vi "마이크로세크 카운터.vi"() -> ()   [LabVIEW 2018]
uses:
  <vilib>/DAQmx/read.llb/DAQmx Read (Counter DBL 1Chan 1Samp).vi
  <vilib>/DAQmx/create/channels.llb/DAQmx Create Channel (CI-Count Edges).vi
  <vilib>/DAQmx/miscellaneous.llb/DAQmx Fill In Error Info.vi
panel:
  out "Elapsed time [s]":dbl
  in  "Input Frequency [Hz]":dbl format="%0.2f"
  out "data 2":dbl caption="데이터" format="%0.2f"
  in  "정지 버튼":bool
  in  "edge":i32(ring)=10280 caption="에지" items=["상승"=10280, "하강"=10171]
  in  "count direction":i32(ring)=10128 caption="카운트 방향" items=["카운트 업"=10128, "카운트 다운"=10124, "외부 컨트롤"=10326]
  in  "initial count":u32 caption="초기 카운트"
  in  "counter":tag caption="카운터"
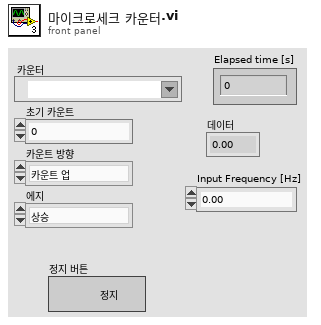
[diagram p1: front panel]
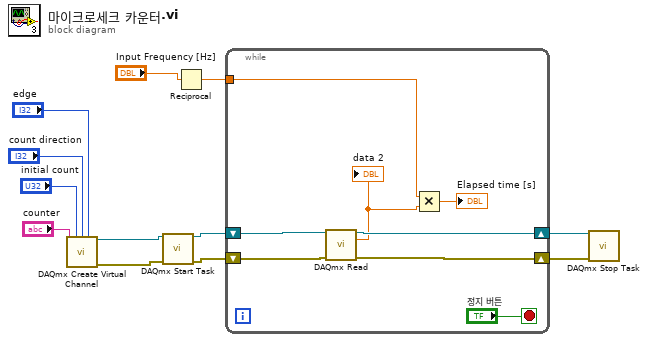
[diagram p0: block diagram]
diagram:
  n1 = call-poly <vilib>:"DAQmx Create Virtual Channel.vi"("initial count"="initial count", "count direction"="count direction", "edge"="edge", "counter"="counter") -> ("task out"=w12:refnum<k21>, "error out"=w11:errorcluster)  [unwired: 10 in]
  n2 = call <vilib>:"DAQmx Start Task.vi"("task/channels in"=w12, "error in"=w11) -> ("task out"=w9:refnum<k21>, "error out"=w10:errorcluster)  [unwired: 12 in]
  n3 = Reciprocal(x="Input Frequency [Hz]") -> (1/x=w1:dbl)
  n4 = while {
    shift-right: [w17] -> w7
    shift-left: w10 -> [w20]
    shift-right: [w18] -> w8
    shift-left: w9 -> [w19]
    tunnel: w1 -> [w14]
    stop <- "정지 버튼" stop-if-true
    n5 = call-poly <vilib>:"DAQmx Read.vi"("task/channels in"=w19, "error in"=w20) -> ("task out"=w18:refnum<k21>, "data"=w15:dbl, "error out"=w17:errorcluster)  [unwired: 11 in]
    "data 2" <- w15
    n6 = Multiply(x=w14, y=w15) -> (x*y=→"Elapsed time [s]":dbl)
  }
  n7 = call <vilib>:"DAQmx Stop Task.vi"("task/channels in"=w8, "error in"=w7) -> ()  [unwired: 12 in, 2 out]
